vi "Test TS Environment Manager API.vi"() -> ()   [LabVIEW 2025]
doc: "TS Environment Manager API Tester."
uses:
  TSDiscovery/TSDiscovery.lvclass
  C:/Users/juanj/Documents/hasbun_wood_engineering/github/Environment-Toolkit-for-TestStand/src/TSDiscovery/TSDiscovery.lvclass
  C:/Users/juanj/Documents/hasbun_wood_engineering/github/Environment-Toolkit-for-TestStand/src/ITSDiscovery/ITSDiscovery.lvclass
  TSDiscovery Mock/TSDiscovery Mock.lvclass
  C:/Users/juanj/Documents/hasbun_wood_engineering/github/Environment-Toolkit-for-TestStand/src/TSDiscovery Mock/TSDiscovery Mock.lvclass
  Process Executor/Process Executor.lvclass
  C:/Users/juanj/Documents/hasbun_wood_engineering/github/Environment-Toolkit-for-TestStand/src/Process Executor/Process Executor.lvclass
  C:/Users/juanj/Documents/hasbun_wood_engineering/github/Environment-Toolkit-for-TestStand/src/IProcess Executor/IProcess Executor.lvclass
  Process Executor Mock/Process Executor Mock.lvclass
  C:/Users/juanj/Documents/hasbun_wood_engineering/github/Environment-Toolkit-for-TestStand/src/Process Executor Mock/Process Executor Mock.lvclass
  TS Environment Manager.lvlib
  <vilib>/Utility/error.llb/DialogType.ctl
  Type Definitions/Architecture--enum.ctl
  Type Definitions/Profile--cluster.ctl
  Type Definitions/TSInstall--cluster.ctl
panel:
  in  "Tab Control":T1(tab)
  in  "Get Installations":bool
  out "Installations":T2[](array[typedef])
  in  "Name":string
  in  "Add Profile":bool
  in  "Get Profile(s)":bool
  out "File":path
  out "Profile(s)":T4[](array[typedef])
  in  "Delete Profile":bool
  in  "File Path":path
  in  "Set Profiles File":bool
  in  "Activate Version":bool
  in  "Environment":path
  in  "Architecture":T3
  in  "Version":string
  in  "Launch Sequence Editor":bool
  in  "Use Mocks":bool
  out "last error":errorcluster
  in  "Show Diagram on Init":bool
  in  "Show Block Diagram":bool
  in  "Stop Module":bool
  in  "Start Module":bool
  in  "Hide Module Panel":bool
  in  "Show Module Panel":bool
  out "Status":string
  out "Module Running?":bool
  # "This VI tests the API for the Module."
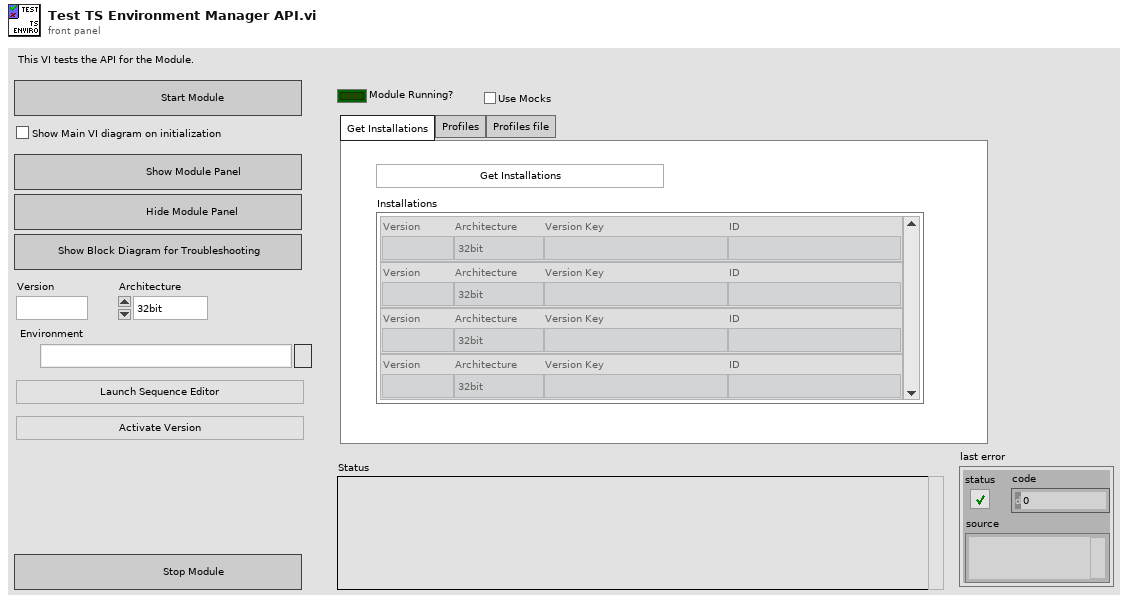
[diagram p1: front panel]
types:
  T1 = enum32{"Get Installations", "Profiles", "Profiles file"}
  T2 = typedef "TSInstall--cluster.ctl" = cluster{"Version":string, "Architecture":T3, "Version Key":string, "ID":string}
  T3 = typedef "Architecture--enum.ctl" = enum16{"32bit", "64bit"}
  T4 = typedef "Profile--cluster.ctl" = cluster{"Name":string, "Version":string, "Architecture":T3, "Environment":path}
  T5 = typedef "TS Environment Manager.lvlib/Broadcast Events--cluster.ctl" = cluster{"Module Did Init":refnum<user-event>, "Status Updated":refnum<user-event>, "Error Reported":refnum<user-event>, "Module Did Stop":refnum<user-event>, "Update Module Execution Status":refnum<user-event>, "Version Activated":refnum<user-event>, "Launched SeqEdit":refnum<user-event>}
  T6 = typedef "DialogType.ctl" = u16
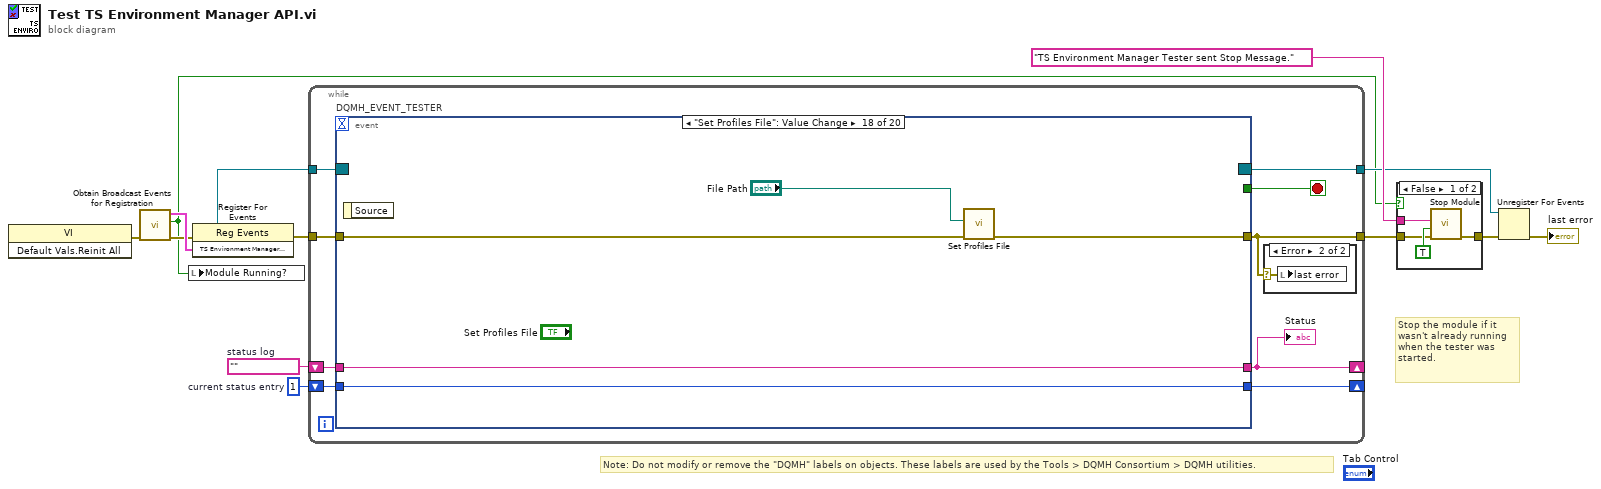
[diagram p0: block diagram]
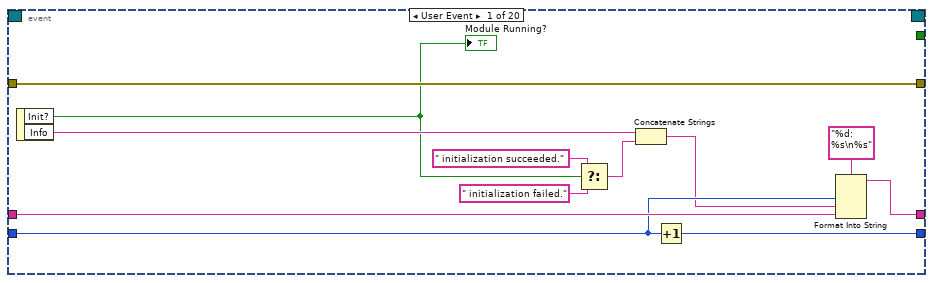
[diagram p4: hidden frame]
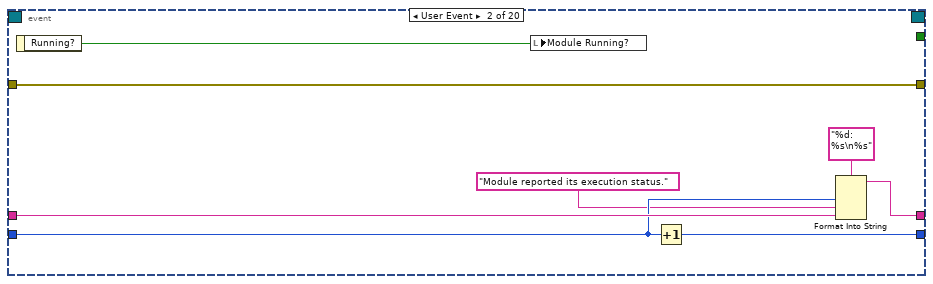
[diagram p5: hidden frame]
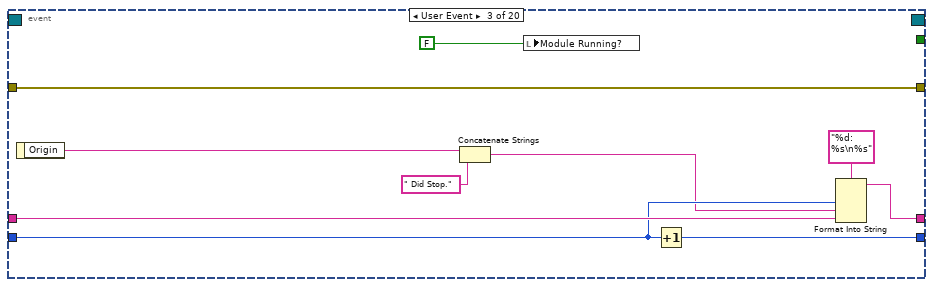
[diagram p6: hidden frame]
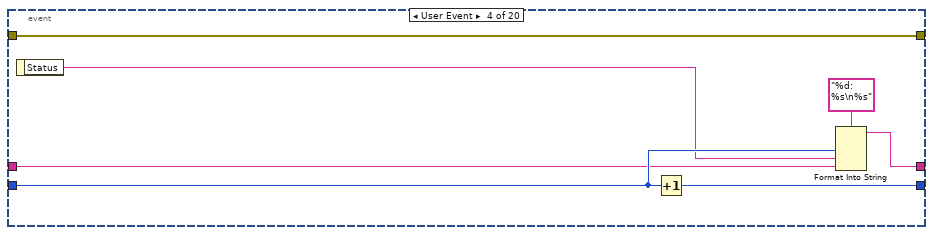
[diagram p7: hidden frame]
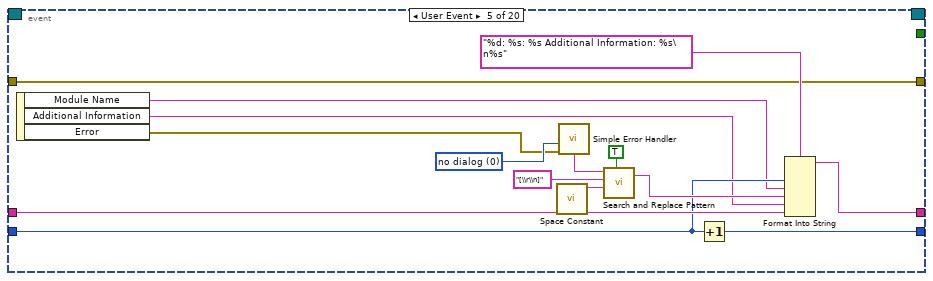
[diagram p8: hidden frame]
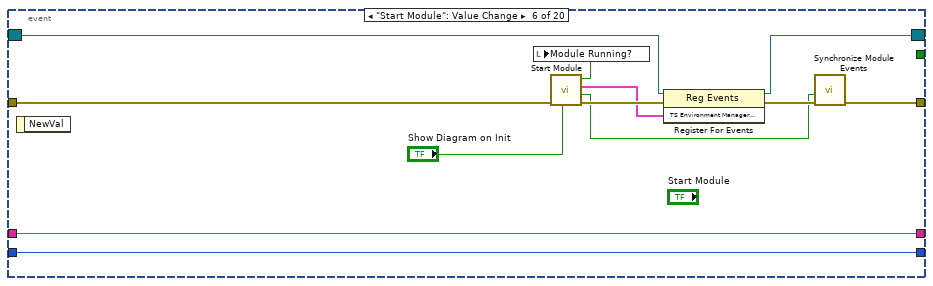
[diagram p9: hidden frame]
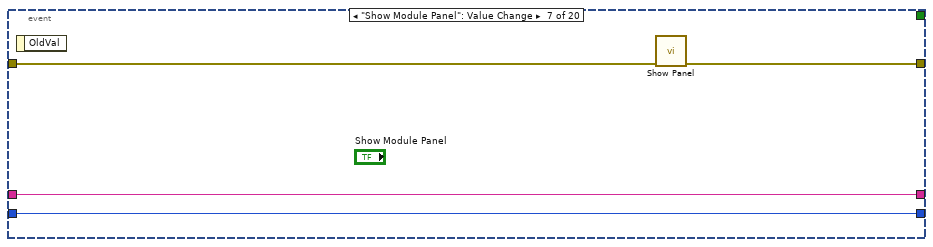
[diagram p10: hidden frame]
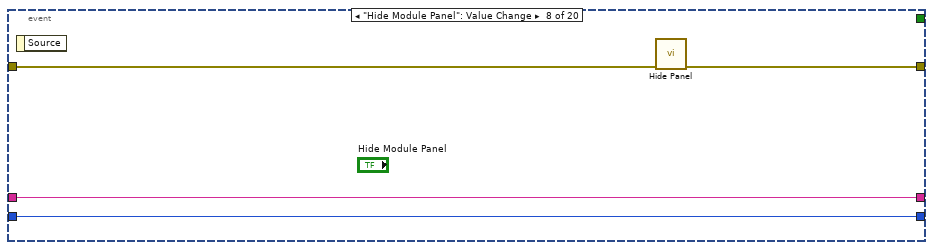
[diagram p11: hidden frame]
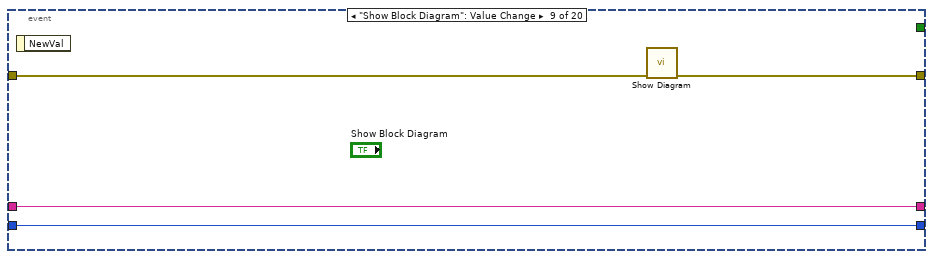
[diagram p12: hidden frame]
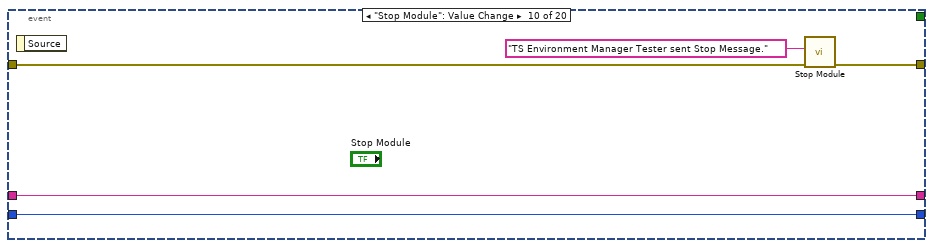
[diagram p13: hidden frame]
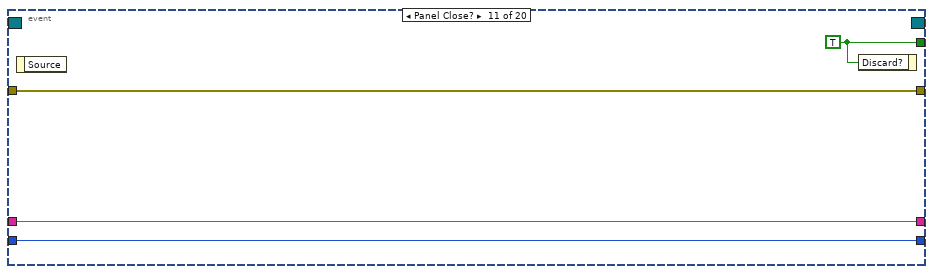
[diagram p14: hidden frame]
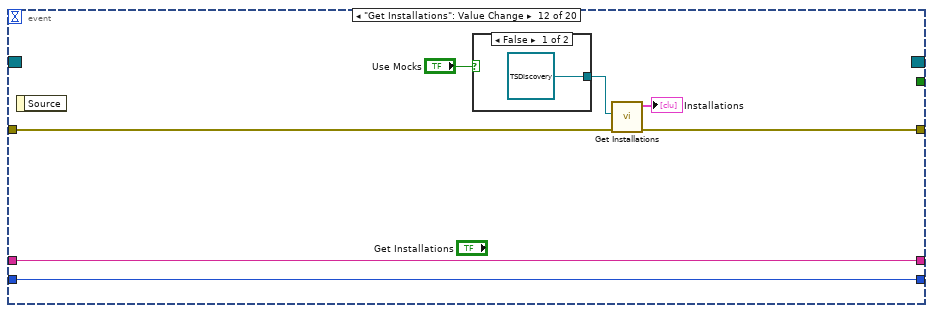
[diagram p15: hidden frame]
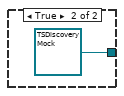
[diagram p16: hidden frame]
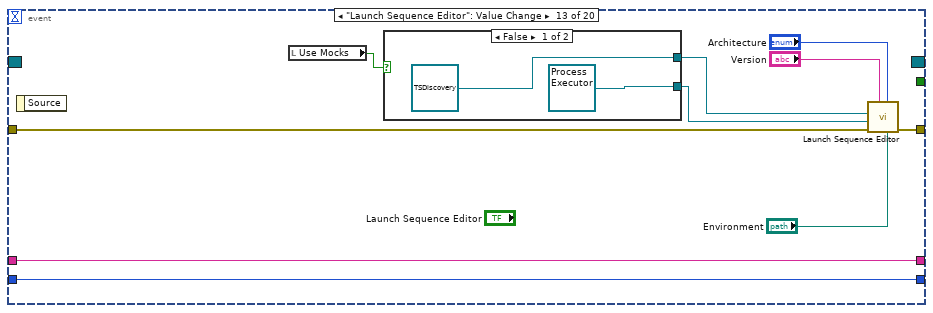
[diagram p17: hidden frame]
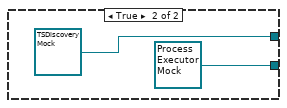
[diagram p18: hidden frame]
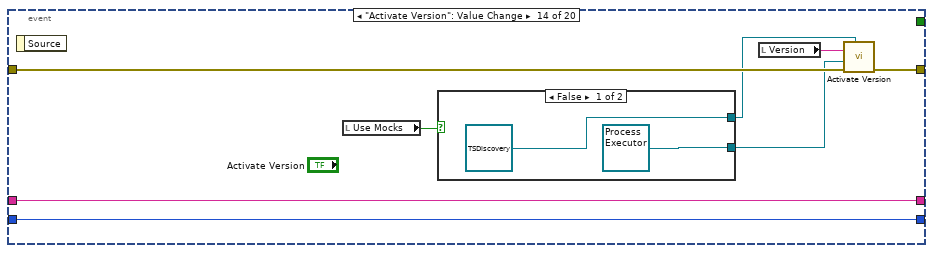
[diagram p19: hidden frame]
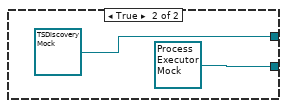
[diagram p20: hidden frame]
diagram:
  w10 = 1  # current status entry
  w11 = ""  # status log
  # "Stop the module if it wasn't already running when the tester was started."
  # "Note: Do not modify or remove the \"DQMH\" labels on objects. These labels are used by the Tools > DQMH Consortium > DQMH utilities."
  n1 = invoke class="VI" method="Default Vals.Reinit All"() -> (error out=w5:errorcluster)  [unwired: 3 in, 2 out]
  n2 = call "Obtain Broadcast Events for Registration.vi"("error in"=w5) -> ("error out"=w4:errorcluster, "Already running?"=w3:bool, "TS Environment Manager Broadcast Events"=w8:T5)  [unwired: 8 in]
  n3 = local write "Module Running?"(w3) -> ()
  n4 = register-events(error in=w4, w8) -> (reference out=w7:refnum<event-registration>, error out=w9:errorcluster)  [unwired: 1 in]
  n5 = while {
    tunnel: w7 -> [w22]
    tunnel: [w14] -> w2
    shift-right: [w18] -> _
    shift-left: w11 -> [w20]
    shift-right: [w19] -> _
    shift-left: w10 -> [w21]
    tunnel: w9 -> [w17]
    tunnel: [w16] -> w6
    stop <- w15 stop-if-true
    n6 = event "DQMH_EVENT_TESTER" shown="[17] \"Set Profiles File\": Value Change" {
      selector: w22 -> [_ _ _ _ _ w81 _ _ _ _ _ _ _ _ _ _ _ _ _ _]
      dyn-events: [_ _ _ _ _ w80 _ _ _ _ _ _ _ _ _ _ _ _ _ _] -> w16
      timeout: _ -> [_ _ _ _ _ _ _ _ _ _ _ _ _ _ _ _ _ _ _ _]
      tunnel: [_ _ _ _ _ _ _ _ _ _ w108 _ _ _ _ _ _ _ _ _] -> w15
      tunnel: [w35 w37 w44 w54 w64 w79 w91 w95 w96 w102 w105 w112 w124 w136 w150 w157 w162 w167 w179 w190] -> w14
      tunnel: w21 -> [w32 w41 w51 w57 w67 w84 w89 w93 w97 w103 w106 w113 w125 w137 w151 w158 w163 w168 w176 w187]
      tunnel: w20 -> [w33 w42 w52 w56 w68 w85 w90 w94 w98 w104 w107 w114 w126 w138 w152 w159 w164 w169 w178 w189]
      tunnel: [w30 w39 w49 w58 w66 w85 w90 w94 w98 w104 w107 w114 w126 w138 w152 w159 w164 w169 w177 w188] -> w18
      tunnel: [w31 w40 w50 w60 w65 w84 w89 w93 w97 w103 w106 w113 w125 w137 w151 w158 w163 w168 w175 w186] -> w19
      tunnel: w17 -> [w35 w37 w44 w54 w64 w78 w88 w92 w99 w100 w105 w115 w127 w139 w153 w160 w165 w170 w179 w190]
      event User Event {
        n7 = event-data() -> ("Init?"=w27:bool, "Info"=w29:string)  [unwired: 1 in]
        "Module Running?" <- w27
        n8 = Select(t=" initialization succeeded.", s=w27, f=" initialization failed.") -> (s? t:f=w24:string)
        n9 = Concatenate Strings(w29, w24) -> (w28:string)
        n10 = Increment(x=w32) -> (x+1=w31:i32)
        n11 = Format Into String(format string="%d: %s\n%s", w32, w28, w33) -> (resulting string=w30:string)  [unwired: 2 in, 1 out]
      }
      event User Event {
        n12 = event-data() -> ("Running?"=w36:bool)  [unwired: 1 in]
        n13 = local write "Module Running?"(w36) -> ()
        n14 = Increment(x=w41) -> (x+1=w40:i32)
        n15 = Format Into String(format string="%d: %s\n%s", w41, "Module reported its execution status.", w42) -> (resulting string=w39:string)  [unwired: 2 in, 1 out]
      }
      event User Event {
        n16 = event-data() -> ("Origin"=w48:string)  [unwired: 1 in]
        n17 = Concatenate Strings(w48, " Did Stop.") -> (w47:string)
        n18 = local write "Module Running?"(FALSE ("Module Did Init?")) -> ()
        n19 = Increment(x=w51) -> (x+1=w50:i32)
        n20 = Format Into String(format string="%d: %s\n%s", w51, w47, w52) -> (resulting string=w49:string)  [unwired: 2 in, 1 out]
      }
      event User Event {
        n21 = event-data() -> ("Status"=w55:string)  [unwired: 1 in]
        n22 = Increment(x=w57) -> (x+1=w60:i32)
        n23 = Format Into String(format string="%d: %s\n%s", w57, w55, w56) -> (resulting string=w58:string)  [unwired: 2 in, 1 out]
      }
      event User Event {
        w69 = T6 0 items=["no dialog", "OK message", "continue or stop message", "OK message + warnings", "continue/stop + warnings"] ("type of dialog (OK msg:1)")
        n24 = event-data() -> ("Module Name"=w63:string, "Additional Information"=w62:string, "Error"=w61:errorcluster)  [unwired: 1 in]
        n25 = call <vilib>:"Space Constant.vi"() -> ("String"=w73:string)
        n26 = call <vilib>:"Simple Error Handler.vi"("type of dialog (OK msg:1)"=w69, "error in (no error)"=w61) -> ("message"=w70:string)  [unwired: 3 in, 4 out]
        n27 = call <vilib>:"Search and Replace Pattern.vi"("string"=w70, "regular expression (\"\")"="[\\r\\n]" ("regular expression (\"\")"), "replace string (\"\")"=w73, "replace all? (F)"=TRUE ("replace all CR/LF with spaces")) -> ("result string"=w71:string)  [unwired: 1 in, 1 out]
        n28 = Increment(x=w67) -> (x+1=w65:i32)
        n29 = Format Into String(format string="%d: %s: %s Additional Information: %s\n%s", w67, w63, w71, w62, w68) -> (resulting string=w66:string)  [unwired: 2 in, 1 out]
      }
      event "Start Module": Value Change {
        n30 = event-data() -> ()  [unwired: 1 in, 1 out]
        n31 = call "Start Module.vi"("Show Main VI Diagram on Init (F)"="Show Diagram on Init", "error in"=w78) -> ("error out"=w86:errorcluster, "Wait for Event Sync?"=w83:bool, "TS Environment Manager Broadcast Events"=w82:T5, "Module Was Already Running?"=w77:bool)  [unwired: 5 in, 1 out]
        n32 = local write "Module Running?"(w77) -> ()
        n33 = register-events(reference=w81, error in=w86, w82) -> (reference out=w80:refnum<event-registration>, error out=w87:errorcluster)
        n34 = call "Synchronize Module Events.vi"("error in"=w87, "Wait for Event Sync?"=w83) -> ("error out"=w79:errorcluster)  [unwired: 9 in]
      }
      event "Show Module Panel": Value Change {
        n35 = event-data() -> ()  [unwired: 1 in, 1 out]
        n36 = call "Show Panel.vi"("error in"=w88) -> ("error out"=w91:errorcluster)  [unwired: 10 in]
      }
      event "Hide Module Panel": Value Change {
        n37 = event-data() -> ()  [unwired: 1 in, 1 out]
        n38 = call "Hide Panel.vi"("error in"=w92) -> ("error out"=w95:errorcluster)  [unwired: 10 in]
      }
      event "Show Block Diagram": Value Change {
        n39 = event-data() -> ()  [unwired: 1 in, 1 out]
        n40 = call "Show Diagram.vi"("error in"=w99) -> ("error out"=w96:errorcluster)  [unwired: 10 in]
      }
      event "Stop Module": Value Change {
        n41 = event-data() -> ()  [unwired: 1 in, 1 out]
        n42 = call "Stop Module.vi"("error in"=w100, "Origin"="TS Environment Manager Tester sent Stop Message.") -> ("error out"=w102:errorcluster)  [unwired: 9 in]
      }
      event Panel Close? {
        w108 = TRUE ("Discard?")
        n43 = event-data() -> ()  [unwired: 1 in, 1 out]
        n44 = event-data("Discard?"=w108) -> ()  [unwired: 1 in, 1 out]
      }
      event "Get Installations": Value Change {
        n45 = event-data() -> ()  [unwired: 1 in, 1 out]
        n46 = case shown="False" "Use Mocks" {
          tunnel: [refnum<class "TSDiscovery.lvclass"> refnum ("TSDiscovery.lvclass") refnum<class "TSDiscovery Mock.lvclass"> refnum ("TSDiscovery Mock.lvclass")] -> w110
          frame False {
          }
          frame True {
          }
        }
        n47 = call "Get Installations.vi"("error in"=w115, "ITSDiscovery.lvclass"=w110) -> ("error out"=w112:errorcluster, "Installations"=→"Installations":T2[])  [unwired: 7 in, 1 out]
      }
      event "Launch Sequence Editor": Value Change {
        n48 = event-data() -> ()  [unwired: 1 in, 1 out]
        n49 = local read "Use Mocks"() -> (w120:bool)
        n50 = case shown="False" w120 {
          tunnel: [refnum<class "Process Executor.lvclass"> refnum ("Process Executor.lvclass") refnum<class "Process Executor Mock.lvclass"> refnum ("Process Executor Mock.lvclass")] -> w119
          tunnel: [refnum<class "TSDiscovery.lvclass"> refnum ("TSDiscovery.lvclass") refnum<class "TSDiscovery Mock.lvclass"> refnum ("TSDiscovery Mock.lvclass")] -> w118
          frame False {
          }
          frame True {
          }
        }
        n51 = call "Launch Sequence Editor.vi"("Environment"="Environment", "Architecture"="Architecture", "Version"="Version", "error in"=w127, "IProcess Executor.lvclass"=w119, "ITSDiscovery.lvclass"=w118) -> ("error out"=w124:errorcluster)  [unwired: 4 in, 1 out]
      }
      event "Activate Version": Value Change {
        n52 = event-data() -> ()  [unwired: 1 in, 1 out]
        n53 = local read "Use Mocks"() -> (w135:bool)
        n54 = case shown="False" w135 {
          tunnel: [refnum<class "Process Executor.lvclass"> refnum ("Process Executor.lvclass") refnum<class "Process Executor Mock.lvclass"> refnum ("Process Executor Mock.lvclass")] -> w133
          tunnel: [refnum<class "TSDiscovery.lvclass"> refnum ("TSDiscovery.lvclass") refnum<class "TSDiscovery Mock.lvclass"> refnum ("TSDiscovery Mock.lvclass")] -> w134
          frame False {
          }
          frame True {
          }
        }
        n55 = local read "Version"() -> (w132:string)
        n56 = call "Activate Version.vi"("ITSDiscovery.lvclass"=w134, "error in"=w139, "IProcess Executor.lvclass"=w133, "Version"=w132) -> ("error out"=w136:errorcluster)  [unwired: 6 in, 1 out]
      }
      event "Add Profile": Value Change {
        n57 = event-data() -> ()  [unwired: 1 in, 1 out]
        n58 = local read "Environment"() -> (w148:path)
        n59 = local read "Architecture"() -> (w147:T3)
        n60 = local read "Version"() -> (w146:string)
        n61 = Bundle By Name(cluster=T4 {"Name"="", "Version"="", "Architecture"=enum."32bit", "Environment"=path ""} ("Profile"), "Name"="Name", "Version"=w146, "Architecture"=w147, "Environment"=w148) -> (w144:T4)
        n62 = call "Add Profile.vi"("error in"=w153, "Profile"=w144) -> ("error out"=w150:errorcluster)  [unwired: 8 in, 1 out]
      }
      event "Get Profile(s)": Value Change {
        n63 = event-data() -> ()  [unwired: 1 in, 1 out]
        n64 = local read "Name"() -> (w156:string)
        n65 = call "Get Profile(s).vi"("error in"=w160, "Name"=w156) -> ("error out"=w157:errorcluster, "File"=→"File":path, "Profile(s)"=→"Profile(s)":T4[])  [unwired: 6 in, 1 out]
      }
      event "Delete Profile": Value Change {
        n66 = event-data() -> ()  [unwired: 1 in, 1 out]
        n67 = local read "Name"() -> (w161:string)
        n68 = call "Delete Profile.vi"("error in"=w165, "Name"=w161) -> ("error out"=w162:errorcluster)  [unwired: 8 in, 1 out]
      }
      event "Set Profiles File": Value Change {
        n69 = event-data() -> ()  [unwired: 1 in, 1 out]
        n70 = call "Set Profiles File.vi"("error in"=w170, "File Path"="File Path") -> ("error out"=w167:errorcluster)  [unwired: 9 in]
      }
      event User Event {
        n71 = event-data() -> ("Version"=w171:string)  [unwired: 1 in, 1 out]
        n72 = Format Into String(format string="Activated Version %s", w171) -> (resulting string=w172:string)  [unwired: 2 in, 1 out]
        n73 = Increment(x=w176) -> (x+1=w175:i32)
        n74 = Format Into String(format string="%d: %s\n%s", w176, w172, w178) -> (resulting string=w177:string)  [unwired: 2 in, 1 out]
      }
      event User Event {
        n75 = event-data() -> ("Version"=w182:string, "Architecture"=w181:T3, "Environment"=w180:path)  [unwired: 1 in, 2 out]
        n76 = Format Into String(format string="Sequence editor launched:\n%s\n%s\n%s", w182, w181, w180) -> (resulting string=w183:string)  [unwired: 2 in, 1 out]
        n77 = Increment(x=w187) -> (x+1=w186:i32)
        n78 = Format Into String(format string="%d: %s\n%s", w187, w183, w189) -> (resulting string=w188:string)  [unwired: 2 in, 1 out]
      }
    }
    "Status" <- w18
    n79 = case shown="Error" w14 {
      selector: w14 -> [_ w23]
      frame No Error {
      }
      frame Error {
        n80 = local write "last error"(w23) -> ()
      }
    }
  }
  n81 = case shown="False" w3 {
    tunnel: [w194 w195] -> w13
    tunnel: "TS Environment Manager Tester sent Stop Message." ("Origin") -> [w193 _]
    tunnel: w2 -> [w191 w195]
    frame False {
      n82 = call "Stop Module.vi"("error in"=w191, "Wait for Module to Stop? (F)"=TRUE ("Wait for Module to stop?"), "Origin"=w193) -> ("error out"=w194:errorcluster)  [unwired: 8 in]
    }
    frame True {
    }
  }
  n83 = Unregister For Events(event registration refnum=w6, error in=w13) -> (error out=→"last error":errorcluster)
